vi "Firmware Wizard Config.vi"(8 "Error In":errorcluster) -> (0 "Error Out":errorcluster)   [LabVIEW 2020, in "LMH-LINX.lvlib"]
doc: "Allow user to configure settings stored in firmware wizard ini."
uses:
  LMH-LINX.lvlib
  <vilib>/Utility/config.llb/Read Key (Path).vi
  <vilib>/Utility/config.llb/Write Key (Path).vi
  <vilib>/Utility/config.llb/NI_LVConfig.lvlib
  Toolbox/LMH-Toolbox.lvlib
panel:
  in  "Generate Firmware Libs":bool
  in  "Arduino Path":path
  in  "Cancel Button":bool
  in  "Save Button":bool
  in  "LINX Firmware Base Path":path
  # "Default Location: <LabVIEW>\\vi.lib\\MakerHub\\LINX\\Firmware\\"
  # "Default Location: <Program Files (x86)>\\Arduino"
  # "If you have the Arduino IDE, fill in the Arduino Path and use the Generate button to Generate the LINX firmware in the Arduino\\libraries folder\nNOTE: This will erase existing LINX firmware in this folder"
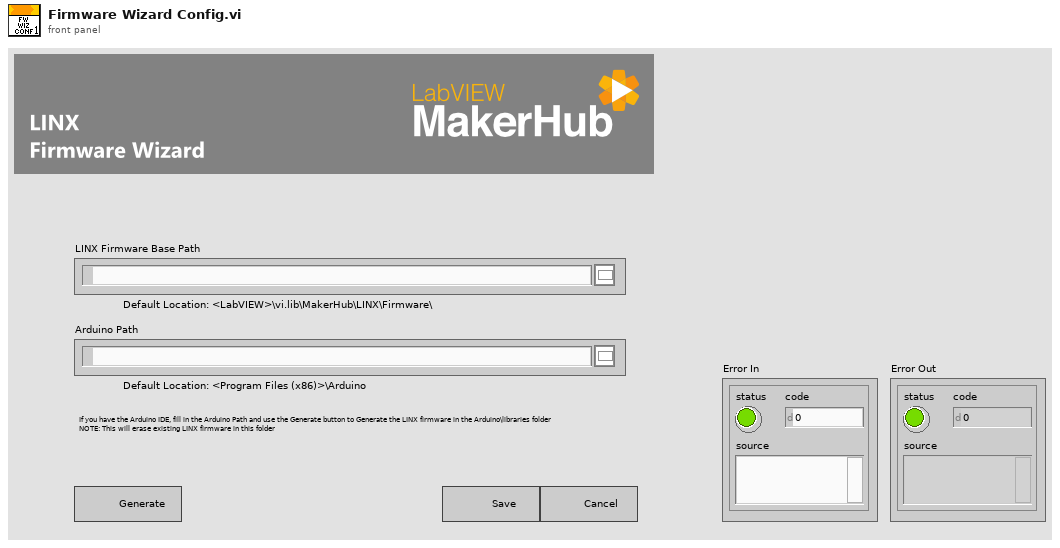
[diagram p1: front panel]
types:
  T1 = typedef "NI_LVConfig.lvlib/Config Data RefNum.ctl" = refnum<k1>
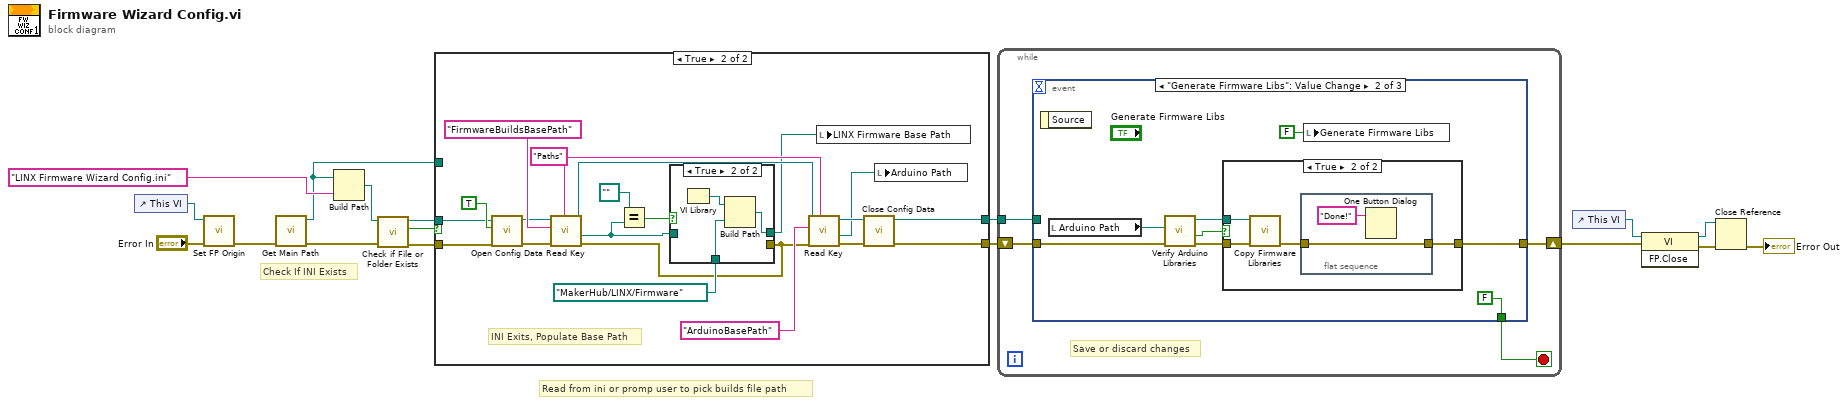
[diagram p0: block diagram]
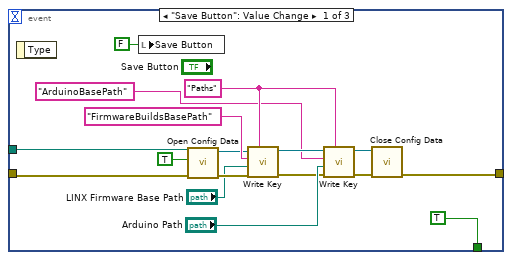
[diagram p2: hidden frame]
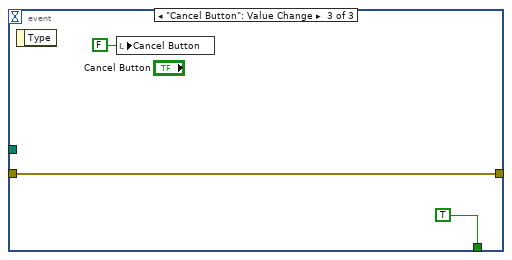
[diagram p4: hidden frame]
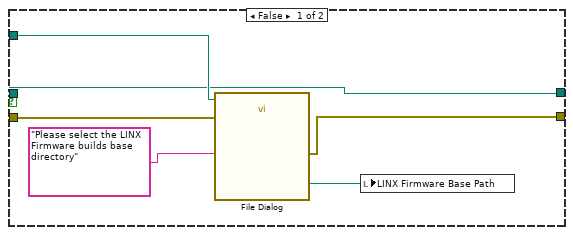
[diagram p5: hidden frame]
diagram:
  # "Read from ini or promp user to pick builds file path"
  # "Check If INI Exists"
  n1 = control-ref of="This VI"() -> (w8:refnum<vi>)
  n2 = call "Set FP Origin.vi"("Error In"="Error In", "VI Ref"=w8) -> ("Error Out"=w1:errorcluster)  [unwired: 9 in]
  n3 = call "Get Main Path.vi"("Error In"=w1) -> ("Error Out"=w16:errorcluster, "Main Dir"=w11:path)  [unwired: 8 in, 1 out]
  n4 = Build Path(base path=w11, name or relative path="LINX Firmware Wizard Config.ini") -> (appended path=w15:path)
  n5 = call <vilib>:"Check if File or Folder Exists.vi"("error in (no error)"=w16, "path"=w15) -> ("error out"=w12:errorcluster, "file or folder exists?"=w13:bool, "dup path"=w14:path)  [unwired: 7 in]
  n6 = case shown="True" w13 {
    tunnel: [w22 w39] -> w10
    tunnel: w14 -> [w20 w38]
    tunnel: w12 -> [w23 w37]
    tunnel: w11 -> [w21 _]
    tunnel: [w20 w36] -> w9
    frame False {
      n7 = call "File Dialog"("start path"=w21, "prompt"="Please select the LINX Firmware builds base directory", "error in"=w23) -> ("selected path"=w19:path, "error out"=w22:errorcluster)  [unwired: 9 in, 2 out]
      n8 = local write "LINX Firmware Base Path"(w19) -> ()
    }
    frame True {
      w34 = "Paths" ("section")
      # "INI Exits, Populate Base Path"
      n9 = call <vilib>:"Open Config Data.vi"("error in (no error)"=w37, "create file if necessary (T)"=TRUE, "configuration file path"=w38) -> ("error out"=w40:errorcluster, "refnum"=w41:T1)  [unwired: 6 in, 1 out]
      n10 = call-poly <vilib>:"Read Key.vi"("section"=w34, "error in (no error)"=w40, "key"="FirmwareBuildsBasePath", "refnum"=w41) -> ("error out"=w27:errorcluster, "value"=w26:path, "refnum out"=w35:T1)  [unwired: 4 in, 1 out]
      n11 = Equal?(x=path "" ("value"), y=w26) -> (x = y?=w24:bool)
      n12 = case shown="True" w24 {
        tunnel: w27 -> [_ _]
        tunnel: path "MakerHub/LINX/Firmware" -> [_ w46]
        tunnel: w26 -> [w44 _]
        tunnel: [w44 w45] -> w28
        frame False {
        }
        frame True {
          n13 = VI Library() -> (path=w47:path)
          n14 = Build Path(base path=w47, name or relative path=w46) -> (appended path=w45:path)
        }
      }
      n15 = call-poly <vilib>:"Read Key.vi"("section"=w34, "error in (no error)"=w27, "key"="ArduinoBasePath", "refnum"=w35) -> ("error out"=w31:errorcluster, "value"=w30:path, "refnum out"=w32:T1)  [unwired: 4 in, 1 out]
      n16 = local write "LINX Firmware Base Path"(w28) -> ()
      n17 = call <vilib>:"Close Config Data.vi"("error in (no error)"=w31, "refnum"=w32) -> ("error out"=w39:errorcluster, "file path"=w36:path)  [unwired: 8 in]
      n18 = local write "Arduino Path"(w30) -> ()
    }
  }
  n19 = while {
    tunnel: w9 -> [w50]
    shift-right: [w49] -> w3
    shift-left: w10 -> [w51]
    stop <- w48 stop-if-true
    # "Save or discard changes"
    n20 = event shown="[1] \"Generate Firmware Libs\": Value Change" {
      selector: _ -> [_ _ _]
      dyn-events: _ -> [_ _ _]
      timeout: _ -> [_ _ _]
      tunnel: w51 -> [w66 w76 w85]
      tunnel: [w61 w69 w85] -> w49
      tunnel: w50 -> [w63 _ _]
      tunnel: [TRUE FALSE TRUE] -> w48
      event "Save Button": Value Change {
        w58 = "Paths" ("section")
        n21 = event-data() -> ()  [unwired: 1 in, 1 out]
        n22 = local write "Save Button"(FALSE ("Save Button")) -> ()
        n23 = call <vilib>:"Open Config Data.vi"("error in (no error)"=w66, "create file if necessary (T)"=TRUE, "configuration file path"=w63) -> ("error out"=w65:errorcluster, "refnum"=w62:T1)  [unwired: 6 in, 1 out]
        n24 = call-poly <vilib>:"Write Key.vi"("section"=w58, "error in (no error)"=w65, "value"="LINX Firmware Base Path", "key"="FirmwareBuildsBasePath", "refnum"=w62) -> ("error out"=w55:errorcluster, "refnum out"=w59:T1)  [unwired: 4 in, 1 out]
        n25 = call-poly <vilib>:"Write Key.vi"("section"=w58, "error in (no error)"=w55, "value"="Arduino Path", "key"="ArduinoBasePath", "refnum"=w59) -> ("error out"=w54:errorcluster, "refnum out"=w53:T1)  [unwired: 4 in, 1 out]
        n26 = call <vilib>:"Close Config Data.vi"("error in (no error)"=w54, "refnum"=w53) -> ("error out"=w61:errorcluster)  [unwired: 8 in, 1 out]
      }
      event "Generate Firmware Libs": Value Change {
        n27 = event-data() -> ()  [unwired: 1 in, 1 out]
        n28 = local read "Arduino Path"() -> (w75:path)
        n29 = call "Verify Arduino Libraries.vi"("Error In"=w76, "Arduino Base Path"=w75) -> ("Error Out"=w73:errorcluster, "Arduino IDE Found?"=w70:bool, "Path to Arduino\\libraries"=w74:path)  [unwired: 6 in, 1 out]
        n30 = case shown="True" w70 {
          tunnel: w74 -> [_ w81]
          tunnel: w73 -> [w77 w80]
          tunnel: [w77 w78] -> w69
          frame False {
          }
          frame True {
            n31 = call "Copy Firmware Libraries.vi"("Error In"=w80, "Library Destination Dir"=w81) -> ("Error Out"=w79:errorcluster)  [unwired: 9 in]
            n32 = flat-sequence {
              tunnel: w79 -> [w83]
              tunnel: [w83] -> w78
              frame #0 {
                n33 = One Button Dialog(message="Done!") -> ()  [unwired: 1 in, 1 out]
              }
            }
          }
        }
        n34 = local write "Generate Firmware Libs"(FALSE ("Generate Firmware Libs")) -> ()
      }
      event "Cancel Button": Value Change {
        n35 = event-data() -> ()  [unwired: 1 in, 1 out]
        n36 = local write "Cancel Button"(FALSE ("Cancel Button")) -> ()
      }
    }
  }
  n37 = control-ref of="This VI"() -> (w4:refnum<vi>)
  n38 = invoke class="VI" method="FP.Close"(reference=w4, error in=w3) -> (reference out=w6:refnum<vi>, error out=w5:errorcluster)  [unwired: 1 in, 1 out]
  n39 = Close Reference(reference=w6, error in (no error)=w5) -> (error out=→"Error Out":errorcluster)
